vi "Create from Subprocess.vi"(8 "error in (no error)":errorcluster, 11 "subprocess":refnum<class "Subprocess.lvclass">) -> (0 "error out":errorcluster, 3 "buffered subprocess":refnum<class "Buffered Subprocess.lvclass">)   [LabVIEW 2020, in "NI_Subprocess.lvlib" / "Buffered Subprocess.lvclass"]
doc: "Construct a Buffered Subprocess by encapsulating a Subprocess."
uses:
  <vilib>/Subprocess/Buffered Subprocess/Buffered Subprocess.lvclass
  <vilib>/Subprocess/Subprocess/Subprocess.lvclass
  <vilib>/Subprocess/Buffered Subprocess/Buffered Subprocess.lvclass/Buffered Subprocess.ctl
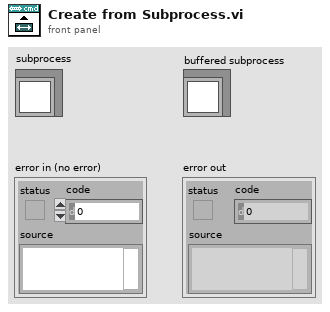
[diagram p1: front panel]
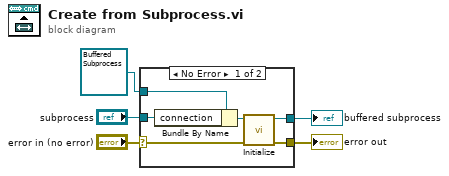
[diagram p0: block diagram]
diagram:
  n1 = case shown="No Error" "error in (no error)" {
    selector: "error in (no error)" -> [w9 w13]
    tunnel: [w8 w13] -> w1
    tunnel: [w7 w12] -> w2
    tunnel: refnum<class "Buffered Subprocess.lvclass"> refnum ("Buffered Subprocess in") -> [w6 w12]
    tunnel: "subprocess" -> [w11 _]
    frame No Error {
      n2 = Bundle By Name(cluster=w6, "connection"=w11) -> (w10:refnum<class "Buffered Subprocess.lvclass">)
      n3 = call-dynamic "Initialize.vi"("error in (no error)"=w9, "subprocess in"=w10) -> ("error out"=w8:errorcluster, "subprocess out"=w7:refnum<class "Buffered Subprocess.lvclass">)  [unwired: 8 in]
    }
    frame Error {
    }
  }
  "error out" <- w1
  "buffered subprocess" <- w2
